vi "MM_WireClass.vi"(8 "error in (no error)":errorcluster, 11 "vi reference":refnum<vi>) -> (0 "error out":errorcluster, 3 "dup VI Refnum":refnum<vi>)   [LabVIEW 2020]
uses:
  <vilib>/Utility/traverseref.llb/TRef TravTarget.ctl
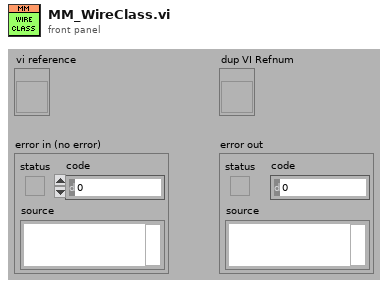
[diagram p1: front panel]
types:
  T1 = typedef "TRef TravTarget.ctl" = enum16{"FP", "BD", "Other"}
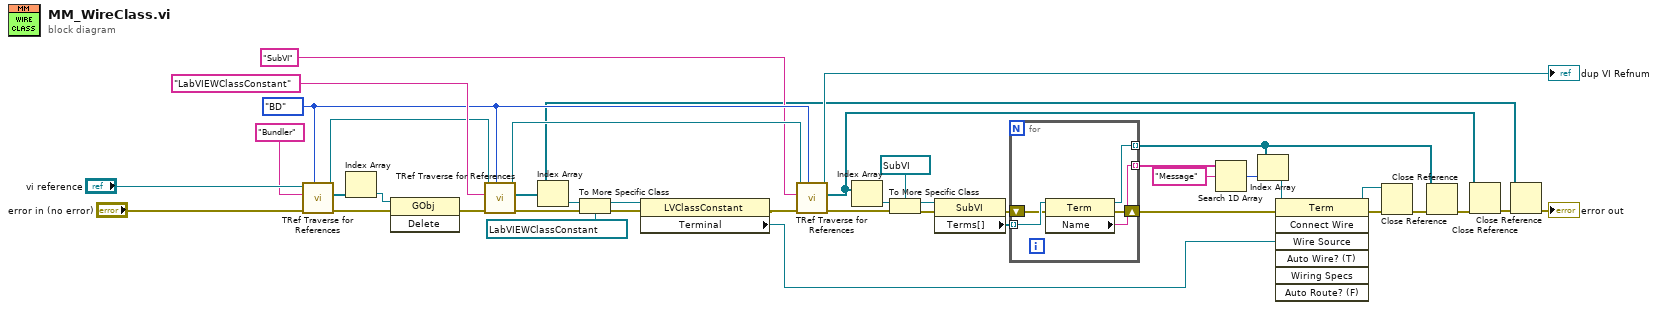
[diagram p0: block diagram]
diagram:
  w31 = TRef_TravTarget."BD" ("Traverse Target")
  n1 = call <vilib>:"TRef Traverse for References.vi"("Traverse Target"=w31, "error in (no error)"="error in (no error)", "Class Name"="Bundler", "VI Refnum"="vi reference") -> ("error out"=w35:errorcluster, "References"=w9:refnum<vi>[], "dup VI Refnum"=w36:refnum<vi>)  [unwired: 4 in, 1 out]
  n2 = Index Array(array=w9) -> (element=w34:refnum<vi>)  [unwired: 1 in]
  n3 = invoke class="GObj" method="Delete"(reference=w34, error in=w35) -> (error out=w33:errorcluster)  [unwired: 1 in, 2 out]
  n4 = call <vilib>:"TRef Traverse for References.vi"("Traverse Target"=w31, "error in (no error)"=w33, "Class Name"="LabVIEWClassConstant", "VI Refnum"=w36) -> ("error out"=w6:errorcluster, "References"=w11:refnum<vi>[], "dup VI Refnum"=w32:refnum<vi>)  [unwired: 4 in, 1 out]
  n5 = Index Array(array=w11) -> (element=w8:refnum<vi>)  [unwired: 1 in]
  n6 = To More Specific Class(target class=refnum<vi> refnum ("element"), reference=w8, error in=w6) -> (specific class reference=w5:refnum<vi>, error out=w4:errorcluster)
  n7 = property class="LVClassConstant"(reference=w5, error in=w4) -> (error out=w3:errorcluster, "Terminal"=w2:refnum<vi>)  [unwired: 1 out]
  n8 = call <vilib>:"TRef Traverse for References.vi"("Traverse Target"=w31, "error in (no error)"=w3, "Class Name"="SubVI", "VI Refnum"=w32) -> ("error out"=w18:errorcluster, "References"=w12:refnum<vi>[], "dup VI Refnum"=→"dup VI Refnum":refnum<vi>)  [unwired: 4 in, 1 out]
  n9 = Index Array(array=w12) -> (element=w29:refnum<vi>)  [unwired: 1 in]
  n10 = To More Specific Class(target class=refnum<vi> refnum ("element"), reference=w29, error in=w18) -> (specific class reference=w25:refnum<vi>, error out=w19:errorcluster)
  n11 = property class="SubVI"(reference=w25, error in=w19) -> (error out=w26:errorcluster, "Terms[]"=w27:refnum<vi>[])  [unwired: 1 out]
  n12 = for {
    tunnel: [w46] -> w24 mode=indexing
    tunnel: w27 -> [w45] mode=indexing
    shift-right: [w43] -> w20
    shift-left: w26 -> [w44]
    tunnel: [w42] -> w14 mode=indexing
    n13 = property class="Term"(reference=w45, error in=w44) -> (reference out=w42:refnum<vi>, error out=w43:errorcluster, "Name"=w46:string)
  }
  n14 = Search 1D Array(1D array=w24, element="Message") -> (index of element=w22:i32)  [unwired: 1 in]
  n15 = Index Array(array=w14, index=w22) -> (element=w21:refnum<vi>)
  n16 = invoke class="Term" method="Connect Wire"(reference=w21, error in=w20, "Wire Source"=w2) -> (reference out=w16:refnum<vi>, error out=w17:errorcluster)  [unwired: 4 in, 5 out]
  n17 = Close Reference(reference=w16, error in (no error)=w17) -> (error out=w15:errorcluster)
  n18 = Close Reference(reference=w14, error in (no error)=w15) -> (error out=w13:errorcluster)
  n19 = Close Reference(reference=w12, error in (no error)=w13) -> (error out=w10:errorcluster)
  n20 = Close Reference(reference=w11, error in (no error)=w10) -> (error out=→"error out":errorcluster)
